vi "主介面.vi"() -> ()   [LabVIEW 2022 SP3]
uses:
  <vilib>/Utility/file.llb/Write Delimited Spreadsheet (string).vi
  <vilib>/httpClient/LabVIEWHTTPClient.lvlib
panel:
  in  "Clean Log":bool
  out "data request times":dbl
  out "SV":dbl
  out "PV":dbl
  in  "ON/OFF":bool
  out "TT-2":dbl
  in  "時間設定":dbl
  out "TT-1":dbl
  out "TT-3":dbl
  out "PT-1":dbl
  out "TT-4":dbl
  out "TT-5":dbl
  out "PT-2":dbl
  out "F14":bool
  out "F13":bool
  out "F12":bool
  out "F11":bool
  out "F10":bool
  out "F9":bool
  out "F8":bool
  out "F1":bool
  out "F2":bool
  out "F3":bool
  out "F4":bool
  out "F5":bool
  out "F6":bool
  out "F7":bool
  out "E1":bool
  out "E5":bool
  out "E4":bool
  out "E3":bool
  out "E2":bool
  out "E6":bool
  out "E7":bool
  out "E8":bool
  out "E9":bool
  out "E10":bool
  out "E11":bool
  out "E15":bool
  out "E14":bool
  out "E13":bool
  out "E12":bool
  out "D1":bool
  out "D2":bool
  out "D3":bool
  out "D4":bool
  out "D5":bool
  out "D6":bool
  out "D7":bool
  out "D8":bool
  out "D9":bool
  out "D10":bool
  out "D11":bool
  out "D12":bool
  out "D13":bool
  out "A0":bool
  in  "stop":bool
  out "C9":bool
  out "C8":bool
  out "C7":bool
  out "C6":bool
  out "C5":bool
  out "C4":bool
  out "C3":bool
  out "C2":bool
  out "C1":bool
  out "B6":bool
  out "B5":bool
  out "B4":bool
  out "B3":bool
  out "B2":bool
  out "B1":bool
  out "A5":bool
  out "A4":bool
  out "A3":bool
  out "A2":bool
  out "A1":bool
  # "S"
  # "HZ"
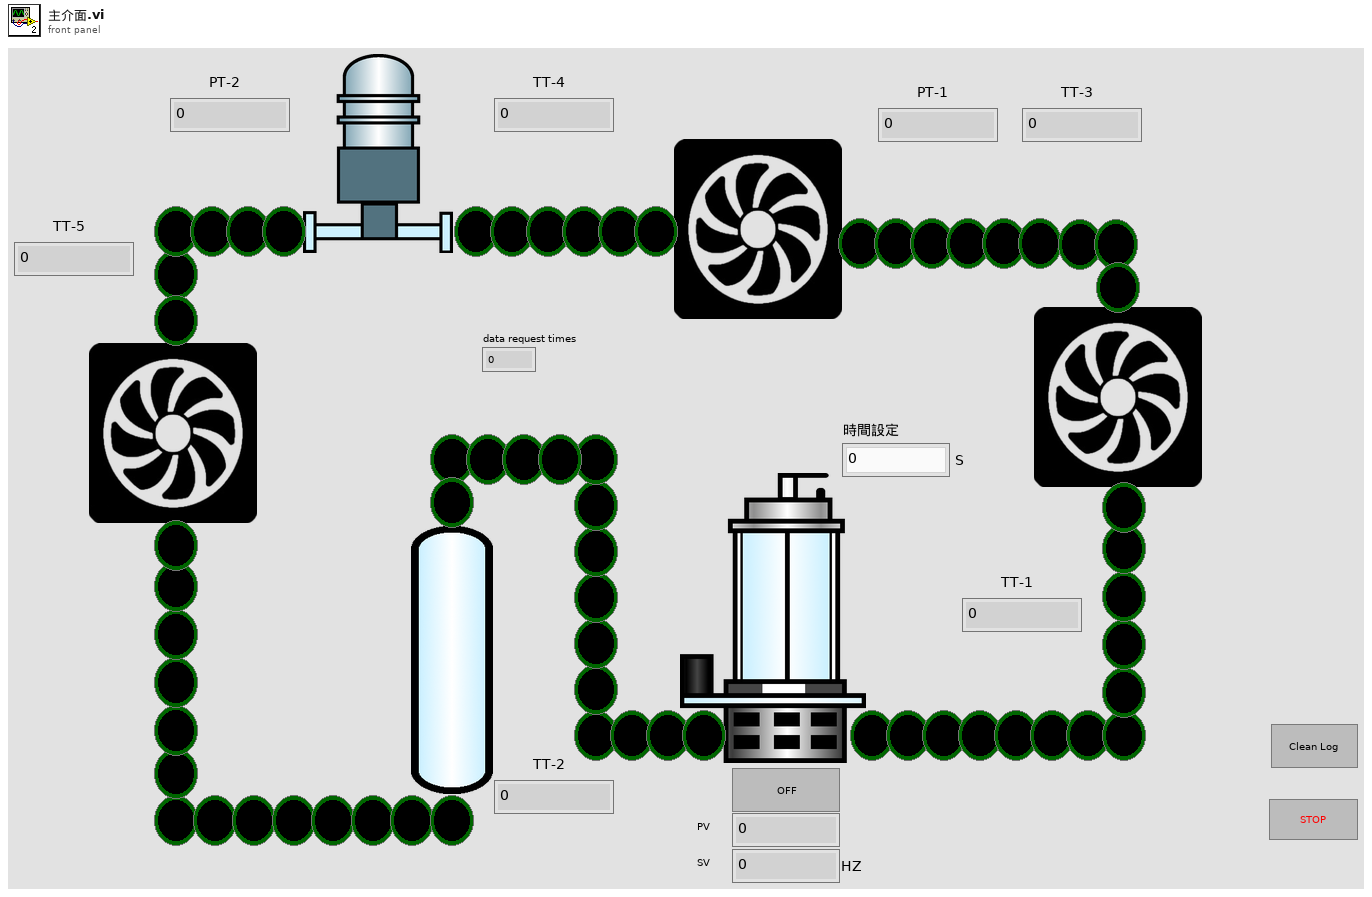
[diagram p1: front panel]
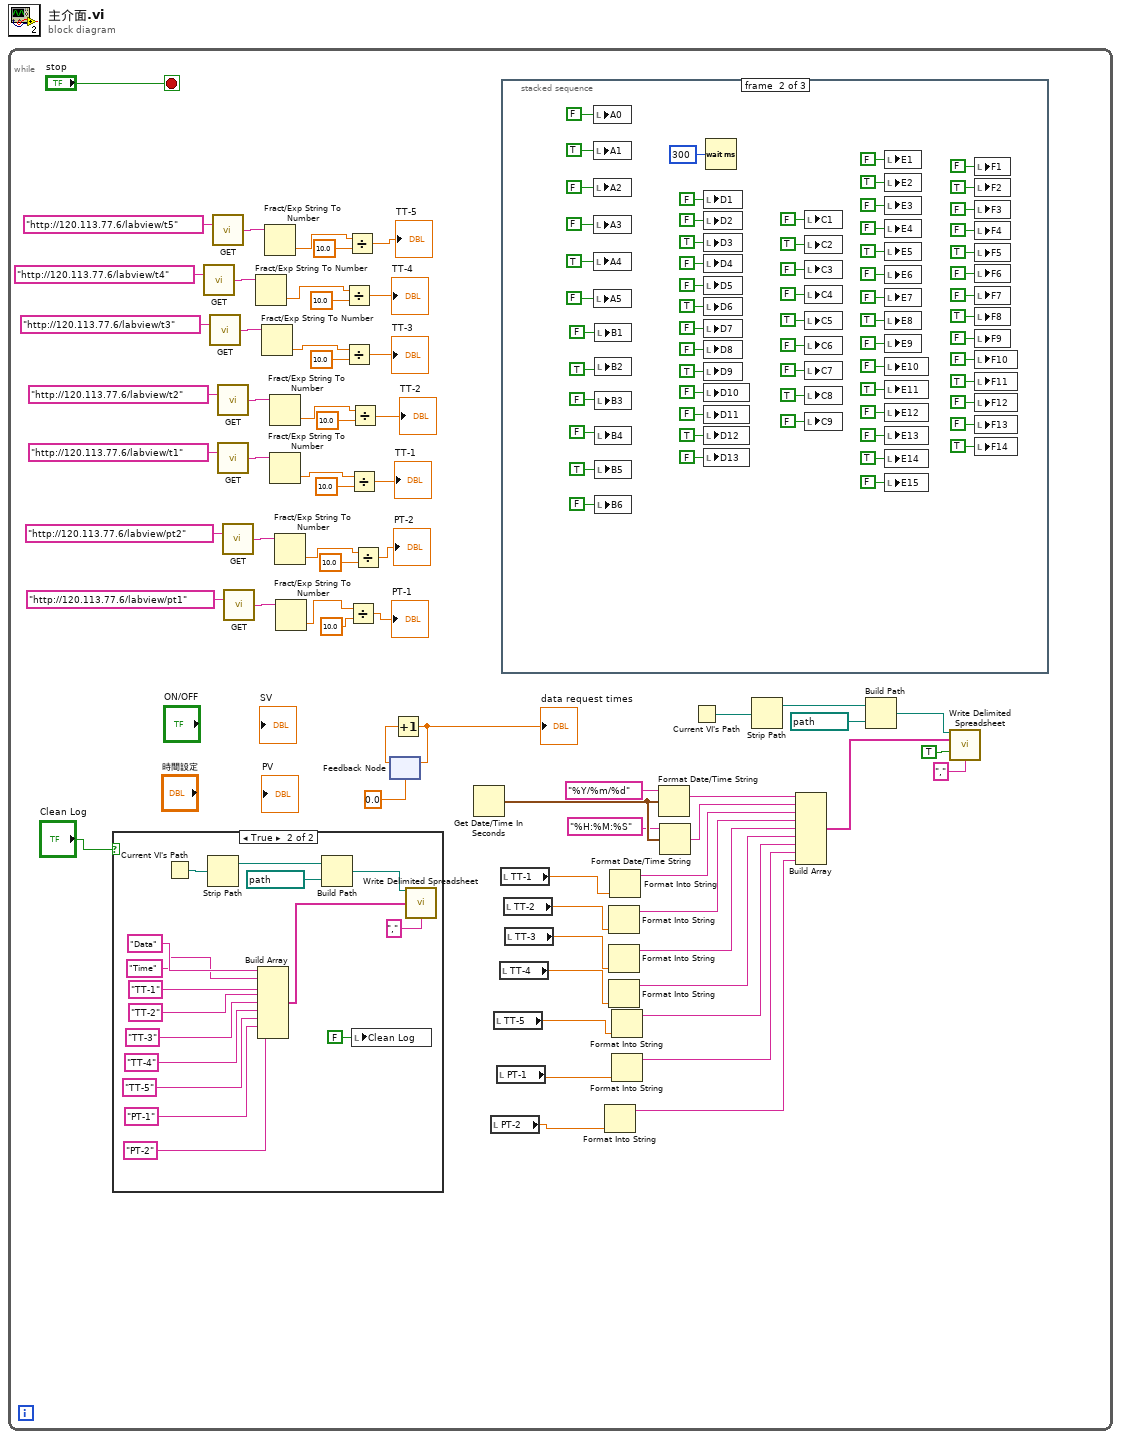
[diagram p0: block diagram]
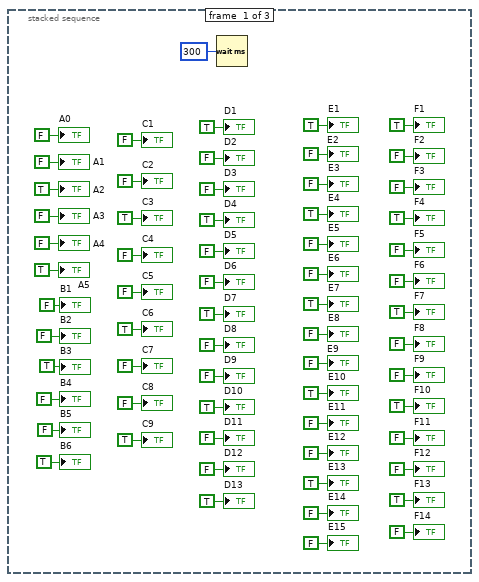
[diagram p3: hidden frame]
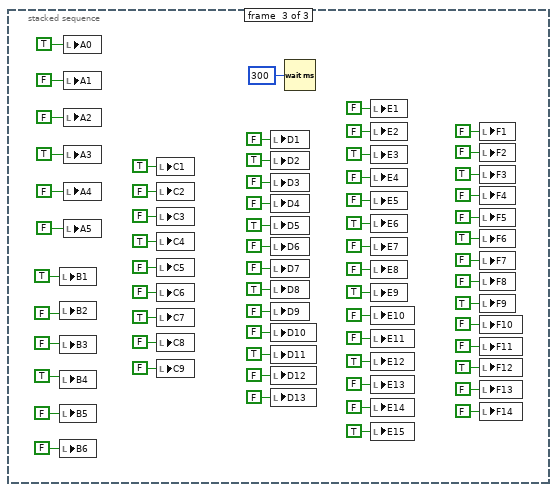
[diagram p4: hidden frame]
diagram:
  n1 = while {
    stop <- "stop" stop-if-true
    n2 = case shown="True" "Clean Log" {
      frame False {
      }
      frame True {
        n3 = Current VI's Path() -> (path=w80:path)
        n4 = Strip Path(path=w80) -> (stripped path=w81:path)  [unwired: 1 out]
        n5 = Build Array("Data" ("time format string (%c)"), "Time" ("time format string (%c)"), "TT-1" ("time format string (%c)"), "TT-2" ("time format string (%c)"), "TT-3" ("time format string (%c)"), "TT-4" ("time format string (%c)"), "TT-5" ("time format string (%c)"), "PT-1" ("time format string (%c)"), "PT-2" ("time format string (%c)")) -> (w79:string[])
        n6 = Build Path(base path=w81, name or relative path=path "溫度.csv") -> (appended path=w82:path)
        n7 = local write "Clean Log"(FALSE ("Clean Log")) -> ()
        n8 = call-poly <vilib>:"Write Delimited Spreadsheet.vi"("file path (dialog if empty)"=w82, "1D data"=w79, "delimiter (\\t)"="," ("delimiter (\\t)")) -> ()  [unwired: 11 in, 2 out]
      }
    }
    n9 = call <vilib>:"GET.vi"("url"="http://120.113.77.6/labview/t4") -> ("body"=w63:string)  [unwired: 11 in, 3 out]
    n10 = call <vilib>:"GET.vi"("url"="http://120.113.77.6/labview/t3") -> ("body"=w60:string)  [unwired: 11 in, 3 out]
    n11 = call <vilib>:"GET.vi"("url"="http://120.113.77.6/labview/t5") -> ("body"=w64:string)  [unwired: 11 in, 3 out]
    n12 = call <vilib>:"GET.vi"("url"="http://120.113.77.6/labview/t2") -> ("body"=w59:string)  [unwired: 11 in, 3 out]
    n13 = call <vilib>:"GET.vi"("url"="http://120.113.77.6/labview/t1") -> ("body"=w56:string)  [unwired: 11 in, 3 out]
    n14 = call <vilib>:"GET.vi"("url"="http://120.113.77.6/labview/pt2") -> ("body"=w55:string)  [unwired: 11 in, 3 out]
    n15 = call <vilib>:"GET.vi"("url"="http://120.113.77.6/labview/pt1") -> ("body"=w52:string)  [unwired: 11 in, 3 out]
    n16 = Fract/Exp String To Number(string=w63) -> (number=w31:dbl)  [unwired: 3 in, 1 out]
    n17 = Fract/Exp String To Number(string=w60) -> (number=w32:dbl)  [unwired: 3 in, 1 out]
    n18 = Fract/Exp String To Number(string=w64) -> (number=w30:dbl)  [unwired: 3 in, 1 out]
    n19 = Fract/Exp String To Number(string=w59) -> (number=w33:dbl)  [unwired: 3 in, 1 out]
    n20 = Fract/Exp String To Number(string=w56) -> (number=w34:dbl)  [unwired: 3 in, 1 out]
    n21 = Fract/Exp String To Number(string=w55) -> (number=w36:dbl)  [unwired: 3 in, 1 out]
    n22 = Fract/Exp String To Number(string=w52) -> (number=w35:dbl)  [unwired: 3 in, 1 out]
    n23 = Divide(x=w31, y=10.0) -> (x/y=→"TT-4":dbl)
    n24 = Divide(x=w32, y=10.0) -> (x/y=→"TT-3":dbl)
    n25 = Divide(x=w30, y=10.0) -> (x/y=→"TT-5":dbl)
    n26 = Divide(x=w35, y=10.0) -> (x/y=→"PT-1":dbl)
    n27 = Divide(x=w34, y=10.0) -> (x/y=→"TT-1":dbl)
    n28 = Divide(x=w33, y=10.0) -> (x/y=→"TT-2":dbl)
    n29 = Divide(x=w36, y=10.0) -> (x/y=→"PT-2":dbl)
    n30 = feedback #1(0.0 ("x")) -> (w49:dbl)
    n31 = Increment(x=w49) -> (x+1=w50:dbl)
    "data request times" <- w50
    n32 = feedback-in #1(w50) -> ()
    n33 = Get Date/Time In Seconds() -> (seconds since 1Jan1904=w26:timestamp)
    n34 = local read "PT-2"() -> (w15:dbl)
    n35 = local read "TT-5"() -> (w13:dbl)
    n36 = local read "PT-1"() -> (w14:dbl)
    n37 = local read "TT-4"() -> (w12:dbl)
    n38 = local read "TT-1"() -> (w16:dbl)
    n39 = stacked-sequence {
      frame #0 {
        n40 = Wait (ms)(milliseconds to wait=u32 300) -> ()  [unwired: 1 out]
        "A2" <- TRUE ("A2")
        "A3" <- FALSE ("A3")
        "A4" <- FALSE ("A4")
        "A5" <- TRUE ("A5")
        "A1" <- FALSE ("A1")
        "B1" <- FALSE
        "B2" <- FALSE
        "B3" <- TRUE
        "B4" <- FALSE
        "B5" <- FALSE
        "B6" <- TRUE
        "C1" <- FALSE ("C1")
        "C2" <- FALSE ("C2")
        "C3" <- TRUE ("C3")
        "C4" <- FALSE ("C4")
        "C5" <- FALSE ("C5")
        "C6" <- TRUE ("C6")
        "C7" <- FALSE ("C7")
        "C8" <- FALSE ("C8")
        "C9" <- TRUE ("C9")
        "A0" <- FALSE ("A1 2")
        "D5" <- FALSE ("D5")
        "D4" <- TRUE ("D4")
        "D3" <- FALSE ("D3")
        "D2" <- FALSE ("D2")
        "D1" <- TRUE ("D1")
        "D6" <- FALSE ("D6")
        "D7" <- TRUE ("D7")
        "D8" <- FALSE ("D8")
        "D9" <- FALSE ("D9")
        "D10" <- TRUE ("D10")
        "D11" <- FALSE ("D11")
        "D12" <- FALSE ("D12")
        "D13" <- TRUE ("D13")
        "F7" <- TRUE ("F7")
        "F6" <- FALSE ("F6")
        "F5" <- FALSE ("F5")
        "F4" <- TRUE ("F4")
        "F3" <- FALSE ("F3")
        "F2" <- FALSE ("F2")
        "F1" <- TRUE ("F1")
        "F8" <- FALSE ("F8")
        "F10" <- TRUE ("F10")
        "F11" <- FALSE ("F11")
        "F12" <- FALSE ("F12")
        "F13" <- TRUE ("F13")
        "F14" <- FALSE ("F14")
        "F9" <- FALSE ("F9")
        "E2" <- FALSE ("E2")
        "E3" <- FALSE ("E3")
        "E1" <- TRUE ("E1")
        "E4" <- TRUE ("E4")
        "E5" <- FALSE ("E5")
        "E12" <- FALSE ("E12")
        "E13" <- TRUE ("E13")
        "E14" <- FALSE ("E14")
        "E15" <- FALSE ("E15")
        "E11" <- FALSE ("E11")
        "E10" <- TRUE ("E10")
        "E9" <- FALSE ("E9")
        "E8" <- FALSE ("E8")
        "E7" <- TRUE ("E7")
        "E6" <- FALSE ("E6")
      }
      frame #1 {
        n41 = local write "A0"(FALSE ("A1 2")) -> ()
        n42 = local write "A1"(TRUE ("A1")) -> ()
        n43 = local write "A2"(FALSE ("A2")) -> ()
        n44 = local write "A3"(FALSE ("A3")) -> ()
        n45 = local write "A4"(TRUE ("A4")) -> ()
        n46 = local write "A5"(FALSE ("A5")) -> ()
        n47 = local write "B1"(FALSE) -> ()
        n48 = local write "B2"(TRUE) -> ()
        n49 = local write "B3"(FALSE) -> ()
        n50 = local write "B4"(FALSE) -> ()
        n51 = local write "B5"(TRUE) -> ()
        n52 = local write "B6"(FALSE) -> ()
        n53 = local write "D1"(FALSE ("D1")) -> ()
        n54 = local write "D2"(FALSE ("D2")) -> ()
        n55 = local write "D3"(TRUE ("D3")) -> ()
        n56 = local write "D4"(FALSE ("D4")) -> ()
        n57 = local write "D5"(FALSE ("D5")) -> ()
        n58 = local write "D6"(TRUE ("D6")) -> ()
        n59 = local write "D7"(FALSE ("D7")) -> ()
        n60 = local write "D8"(FALSE ("D8")) -> ()
        n61 = local write "D9"(TRUE ("D9")) -> ()
        n62 = local write "D10"(FALSE ("D10")) -> ()
        n63 = local write "D11"(FALSE ("D11")) -> ()
        n64 = local write "D12"(TRUE ("D12")) -> ()
        n65 = local write "D13"(FALSE ("D13")) -> ()
        n66 = Wait (ms)(milliseconds to wait=u32 300) -> ()  [unwired: 1 out]
        n67 = local write "C1"(FALSE ("C1")) -> ()
        n68 = local write "C2"(TRUE ("C2")) -> ()
        n69 = local write "C3"(FALSE ("C3")) -> ()
        n70 = local write "C4"(FALSE ("C4")) -> ()
        n71 = local write "C5"(TRUE ("C5")) -> ()
        n72 = local write "C6"(FALSE ("C6")) -> ()
        n73 = local write "C7"(FALSE ("C7")) -> ()
        n74 = local write "C8"(TRUE ("C8")) -> ()
        n75 = local write "C9"(FALSE ("C9")) -> ()
        n76 = local write "E1"(FALSE ("E1")) -> ()
        n77 = local write "E2"(TRUE ("E2")) -> ()
        n78 = local write "E3"(FALSE ("E3")) -> ()
        n79 = local write "E4"(FALSE ("E4")) -> ()
        n80 = local write "E5"(TRUE ("E5")) -> ()
        n81 = local write "E6"(FALSE ("E6")) -> ()
        n82 = local write "E7"(FALSE ("E7")) -> ()
        n83 = local write "E8"(TRUE ("E8")) -> ()
        n84 = local write "E9"(FALSE ("E9")) -> ()
        n85 = local write "E10"(FALSE ("E10")) -> ()
        n86 = local write "E11"(TRUE ("E11")) -> ()
        n87 = local write "E12"(FALSE ("E12")) -> ()
        n88 = local write "E13"(FALSE ("E13")) -> ()
        n89 = local write "E14"(TRUE ("E14")) -> ()
        n90 = local write "E15"(FALSE ("E15")) -> ()
        n91 = local write "F1"(FALSE ("F1")) -> ()
        n92 = local write "F2"(TRUE ("F2")) -> ()
        n93 = local write "F3"(FALSE ("F3")) -> ()
        n94 = local write "F4"(FALSE ("F4")) -> ()
        n95 = local write "F5"(TRUE ("F5")) -> ()
        n96 = local write "F6"(FALSE ("F6")) -> ()
        n97 = local write "F7"(FALSE ("F7")) -> ()
        n98 = local write "F8"(TRUE ("F8")) -> ()
        n99 = local write "F9"(FALSE ("F9")) -> ()
        n100 = local write "F10"(FALSE ("F10")) -> ()
        n101 = local write "F11"(TRUE ("F11")) -> ()
        n102 = local write "F12"(FALSE ("F12")) -> ()
        n103 = local write "F13"(FALSE ("F13")) -> ()
        n104 = local write "F14"(TRUE ("F14")) -> ()
      }
      frame #2 {
        n105 = local write "B1"(TRUE) -> ()
        n106 = local write "B2"(FALSE) -> ()
        n107 = local write "B3"(FALSE) -> ()
        n108 = local write "B4"(TRUE) -> ()
        n109 = local write "B5"(FALSE) -> ()
        n110 = local write "B6"(FALSE) -> ()
        n111 = local write "A0"(TRUE ("A1 2")) -> ()
        n112 = local write "A1"(FALSE ("A1")) -> ()
        n113 = local write "A2"(FALSE ("A2")) -> ()
        n114 = local write "A3"(TRUE ("A3")) -> ()
        n115 = local write "A4"(FALSE ("A4")) -> ()
        n116 = local write "A5"(FALSE ("A5")) -> ()
        n117 = local write "C1"(TRUE ("C1")) -> ()
        n118 = local write "C2"(FALSE ("C2")) -> ()
        n119 = local write "C3"(FALSE ("C3")) -> ()
        n120 = local write "C4"(TRUE ("C4")) -> ()
        n121 = local write "C5"(FALSE ("C5")) -> ()
        n122 = local write "C6"(FALSE ("C6")) -> ()
        n123 = local write "C7"(TRUE ("C7")) -> ()
        n124 = local write "C8"(FALSE ("C8")) -> ()
        n125 = local write "C9"(FALSE ("C9")) -> ()
        n126 = local write "D1"(FALSE ("D1")) -> ()
        n127 = local write "D2"(TRUE ("D2")) -> ()
        n128 = local write "D3"(FALSE ("D3")) -> ()
        n129 = local write "D4"(FALSE ("D4")) -> ()
        n130 = local write "D5"(TRUE ("D5")) -> ()
        n131 = local write "D6"(FALSE ("D6")) -> ()
        n132 = local write "D7"(FALSE ("D7")) -> ()
        n133 = local write "D8"(TRUE ("D8")) -> ()
        n134 = local write "D9"(FALSE ("D9")) -> ()
        n135 = local write "D10"(FALSE ("D10")) -> ()
        n136 = local write "D11"(TRUE ("D11")) -> ()
        n137 = local write "D12"(FALSE ("D12")) -> ()
        n138 = local write "D13"(FALSE ("D13")) -> ()
        n139 = Wait (ms)(milliseconds to wait=u32 300) -> ()  [unwired: 1 out]
        n140 = local write "E1"(FALSE ("E1")) -> ()
        n141 = local write "E2"(FALSE ("E2")) -> ()
        n142 = local write "E3"(TRUE ("E3")) -> ()
        n143 = local write "E4"(FALSE ("E4")) -> ()
        n144 = local write "E5"(FALSE ("E5")) -> ()
        n145 = local write "E6"(TRUE ("E6")) -> ()
        n146 = local write "E7"(FALSE ("E7")) -> ()
        n147 = local write "E8"(FALSE ("E8")) -> ()
        n148 = local write "E9"(TRUE ("E9")) -> ()
        n149 = local write "E10"(FALSE ("E10")) -> ()
        n150 = local write "E11"(FALSE ("E11")) -> ()
        n151 = local write "E12"(TRUE ("E12")) -> ()
        n152 = local write "E13"(FALSE ("E13")) -> ()
        n153 = local write "E14"(FALSE ("E14")) -> ()
        n154 = local write "E15"(TRUE ("E15")) -> ()
        n155 = local write "F1"(FALSE ("F1")) -> ()
        n156 = local write "F2"(FALSE ("F2")) -> ()
        n157 = local write "F3"(TRUE ("F3")) -> ()
        n158 = local write "F4"(FALSE ("F4")) -> ()
        n159 = local write "F5"(FALSE ("F5")) -> ()
        n160 = local write "F6"(TRUE ("F6")) -> ()
        n161 = local write "F7"(FALSE ("F7")) -> ()
        n162 = local write "F8"(FALSE ("F8")) -> ()
        n163 = local write "F9"(TRUE ("F9")) -> ()
        n164 = local write "F10"(FALSE ("F10")) -> ()
        n165 = local write "F11"(FALSE ("F11")) -> ()
        n166 = local write "F12"(TRUE ("F12")) -> ()
        n167 = local write "F13"(FALSE ("F13")) -> ()
        n168 = local write "F14"(FALSE ("F14")) -> ()
      }
    }
    n169 = local read "TT-2"() -> (w10:dbl)
    n170 = local read "TT-3"() -> (w11:dbl)
    n171 = Format Into String(w15) -> (resulting string=w3:string)  [unwired: 3 in, 1 out]
    n172 = Format Into String(w10) -> (resulting string=w8:string)  [unwired: 3 in, 1 out]
    n173 = Format Into String(w11) -> (resulting string=w7:string)  [unwired: 3 in, 1 out]
    n174 = Format Into String(w12) -> (resulting string=w6:string)  [unwired: 3 in, 1 out]
    n175 = Format Into String(w16) -> (resulting string=w9:string)  [unwired: 3 in, 1 out]
    n176 = Format Into String(w13) -> (resulting string=w5:string)  [unwired: 3 in, 1 out]
    n177 = Format Into String(w14) -> (resulting string=w4:string)  [unwired: 3 in, 1 out]
    n178 = Format Date/Time String(time format string (%c)="%Y/%m/%d", seconds (now)=w26) -> (date/time string=w18:string)  [unwired: 1 in]
    n179 = Format Date/Time String(time format string (%c)="%H:%M:%S", seconds (now)=w26) -> (date/time string=w17:string)  [unwired: 1 in]
    n180 = Current VI's Path() -> (path=w24:path)
    n181 = Strip Path(path=w24) -> (stripped path=w23:path)  [unwired: 1 out]
    n182 = Build Array(w18, w17, w9, w8, w7, w6, w5, w4, w3) -> (w2:string[])
    n183 = Build Path(base path=w23, name or relative path=path "溫度.csv") -> (appended path=w21:path)
    n184 = call-poly <vilib>:"Write Delimited Spreadsheet.vi"("file path (dialog if empty)"=w21, "1D data"=w2, "append to file? (new file:F)"=TRUE, "delimiter (\\t)"="," ("delimiter (\\t)")) -> ()  [unwired: 10 in, 2 out]
  }
